vi "image picker.vi"(5 "compactnessMax":dbl=0.5 format="%#_13g", 7 "compactnessMin":dbl=0.30000001192092896 format="%#_13g", 8 "error in":errorcluster, 10 "rgb constants":T1, 11 "Image In":T2) -> (0 "error out":errorcluster, 2 "report":dbl[](array[numeric]), 3 "Image Out":T2)   [LabVIEW 2015]
uses:
  <vilib>/vision/Image Controls.llb/IMAQ Image.ctl
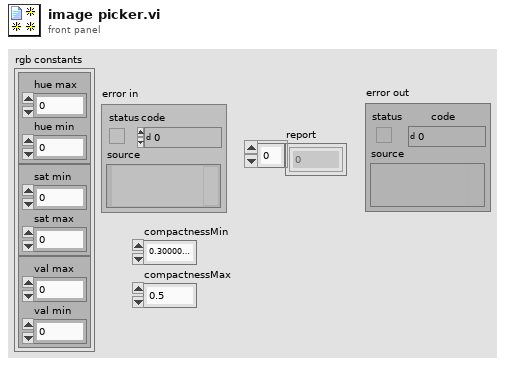
[diagram p1: front panel]
types:
  T1 = cluster{cluster{"hue max":dbl, "hue min":dbl}, cluster{"sat min":dbl, "sat max":dbl}, cluster{"val max":dbl, "val min":dbl}}
  T2 = typedef "IMAQ Image.ctl" = refnum<image>
  T3 = cluster{"Left":i32, "Top":i32, "Right":i32, "Bottom":i32}
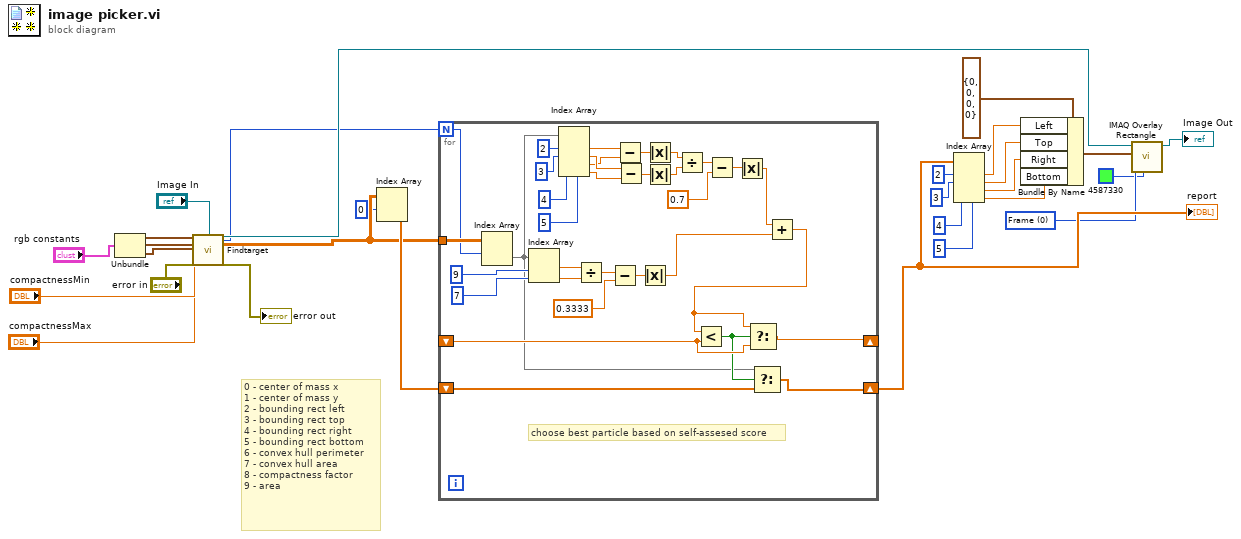
[diagram p0: block diagram]
diagram:
  w9 = u32 0 items=["Frame", "Fill", "Highlight"] ("Drawing Mode (Frame)")
  # "0 - center of mass x\n1 - center of mass y\n2 - bounding rect left\n3 - bounding rect top\n4 - bounding rect right\n5 - bounding rect bottom\n6 - convex hull perimeter\n7 - convex hull area\n8 - compactness factor\n9 - area"
  n1 = Unbundle("rgb constants") -> (w24:cluster{"hue max":dbl, "hue min":dbl}, w23:cluster{"sat min":dbl, "sat max":dbl}, w22:cluster{"val max":dbl, "val min":dbl})
  n2 = call "Findtarget.vi"("Image In"="Image In", "Red or Hue Range (Color Threshold 1)"=w24, "Green or Sat Range (Color Threshold 1)"=w23, "Blue or Luma or Val or Inten Range (Color Threshold 1)"=w22, "compactnessMin"="compactnessMin", "compactnessMax"="compactnessMax", "error in"="error in") -> ("Image Out"=w10:T2, "Number of Particles (Particle Analysis 1)"=w3:i32, "Particle Measurements (Pixels) (Particle Analysis 1)"=w5:dbl[][], "error out"=→"error out":errorcluster)  [unwired: 17 in]
  n3 = Index Array(array=w5, index (row)=0) -> (element=w6:dbl[])  [unwired: 1 in]
  n4 = for {
    N: w3 -> [w60]
    shift-right: [w30] -> w19
    shift-left: w6 -> [w31]
    tunnel: w5 -> [w61]
    shift-right: [w33] -> _
    shift-left: _ -> [w34]
    # "choose best particle based on self-assesed score"
    n5 = Index Array(array=w61, index (row)=w60) -> (element=w29:dbl[])  [unwired: 1 in]
    n6 = Index Array(array=w29, index #1=9 ("index"), index #2=7 ("index")) -> (element #1=w56:dbl, element #2=w57:dbl)
    n7 = Index Array(array=w29, index #1=2 ("index"), index #2=3 ("index"), index #3=4 ("index"), index #4=5 ("index")) -> (element #1=w48:dbl, element #2=w47:dbl, element #3=w45:dbl, element #4=w46:dbl)
    n8 = Divide(x=w56, y=w57) -> (x/y=w55:dbl)
    n9 = Subtract(x=w55, y=0.3333) -> (x-y=w53:dbl)
    n10 = Subtract(x=w48, y=w45) -> (x-y=w44:dbl)
    n11 = Subtract(x=w47, y=w46) -> (x-y=w43:dbl)
    n12 = Absolute Value(x=w53) -> (abs(x)=w36:dbl)
    n13 = Absolute Value(x=w44) -> (abs(x)=w42:dbl)
    n14 = Absolute Value(x=w43) -> (abs(x)=w41:dbl)
    n15 = Divide(x=w42, y=w41) -> (x/y=w40:dbl)
    n16 = Subtract(x=w40, y=0.7) -> (x-y=w38:dbl)
    n17 = Absolute Value(x=w38) -> (abs(x)=w37:dbl)
    n18 = Add(x=w37, y=w36) -> (x+y=w35:dbl)
    n19 = Less?(x=w35, y=w34) -> (x < y?=w32:bool)
    n20 = Select(t=w35, s=w32, f=w34) -> (s? t:f=w33:dbl)
    n21 = Select(t=w29, s=w32, f=w31) -> (s? t:f=w30:dbl[])
  }
  "report" <- w19
  n22 = Index Array(array=w19, index #1=2 ("index"), index #2=3 ("index"), index #3=4 ("index"), index #4=5 ("index")) -> (element #1=w14:dbl, element #2=w13:dbl, element #3=w12:dbl, element #4=w11:dbl)
  n23 = Bundle By Name(cluster=T3 {"Left"=0, "Top"=0, "Right"=0, "Bottom"=0} ("Rectangle"), "Left"=w14, "Top"=w13, "Right"=w12, "Bottom"=w11) -> (w21:T3)
  n24 = call "IMAQ Overlay Rectangle"("Color"=u32 4587330, "Drawing Mode (Frame)"=w9, "Rectangle"=w21, "Image"=w10) -> ("Image Out"=→"Image Out":T2)  [unwired: 6 in, 1 out]
